vi "camelCase Converter.vi"(4 "Input string":string) -> (1 "Output string":string)   [LabVIEW 2025, in "Name Formatter.lvlib"]
doc: "Description:\nTransforms a text with words separated by spaces into <b>camelCase</b>. The first word is lowercase, and each subsequent word starts with an uppercase letter, with no spaces in between.\n\nExample:\nInput -> hello cruel cruel\nOutput -> helloCruelWorld\n\nRequirements:\nThe input must contain spaces. Without spaces, this conversion cannot be applied."
uses:
  Name Formatter.lvlib
panel:
  # "text with spaces"
  # "CamelCase"
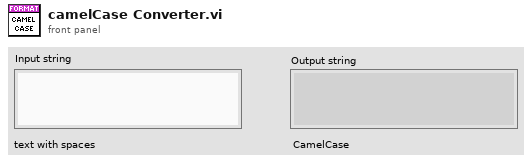
[diagram p1: front panel]
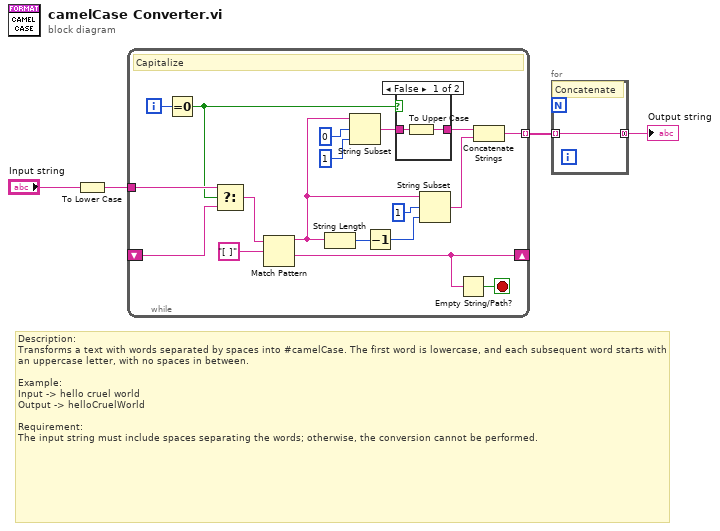
[diagram p0: block diagram]
diagram:
  # "Description:\nTransforms a text with words separated by spaces into #camelCase. The first word is lowercase, and each subsequent word starts with an uppercase letter, with no spaces in between.\n\nExample:\nInput -> hello cruel world\nOutput -> helloCruelWorld\n\nRequirement:\nThe input string must include spaces separating the words; otherwise, the conversion cannot be performed."
  n1 = To Lower Case(string="Input string") -> (all lower case string=w3:string)
  n2 = while {
    tunnel: w3 -> [w21]
    tunnel: [w11] -> w4 mode=indexing
    shift-right: [w18] -> _
    shift-left: _ -> [w19]
    i -> [w9]
    stop <- w17 stop-if-true
    # "Capitalize"
    n3 = Equal To 0?(x=w9) -> (x = 0?=w5:bool)
    n4 = Select(t=w21, s=w5, f=w19) -> (s? t:f=w20:string)
    n5 = Match Pattern(string=w20, regular expression="[ ]") -> (before substring=w10:string, after substring=w18:string)  [unwired: 1 in, 2 out]
    n6 = String Length(string=w10) -> (length=w15:i32)
    n7 = String Subset(string=w10, offset (0)=0, length (rest)=1 ("length (rest)")) -> (substring=w7:string)
    n8 = Decrement(x=w15) -> (x-1=w14:i32)
    n9 = case shown="False" w5 {
      tunnel: [w24 w25] -> w13
      tunnel: w7 -> [w23 w25]
      frame False {
        n10 = To Upper Case(1:w23) -> (0:w24:string)
      }
      frame True {
      }
    }
    n11 = String Subset(string=w10, offset (0)=1, length (rest)=w14) -> (substring=w12:string)
    n12 = Empty String/Path?(string/path=w18) -> (empty?=w17:bool)
    n13 = Concatenate Strings(w13, w12) -> (w11:string)
  }
  n14 = for {
    tunnel: w4 -> [w26] mode=indexing
    tunnel: [w26] -> w1 mode=concatenating
    # "Concatenate"
  }
  "Output string" <- w1
